vi "pop_integer_array.vi"(8 "error in (no error)":errorcluster, 11 "Lua in":refnum<class "Lua.lvclass">) -> (0 "error out":errorcluster, 2 "value":i64[](array[numeric]), 3 "Lua out":refnum<class "Lua.lvclass">)   [LabVIEW 2020, in "Lua for LabVIEW.lvlib" / "Lua.lvclass"]
doc: "Pop a numeric value from the stack."
uses:
  Lua.lvclass
  Lua.lvclass/Lua.ctl
  lib/lua.dll/lua.dll.lvlib
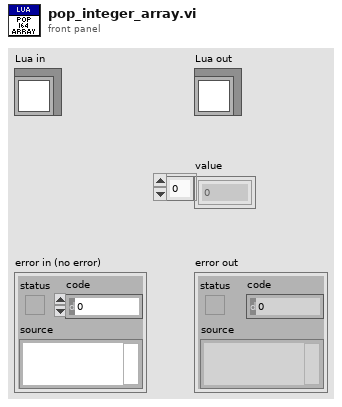
[diagram p1: front panel]
types:
  T1 = typedef "lua.dll.lvlib/lua_types.ctl" = i32
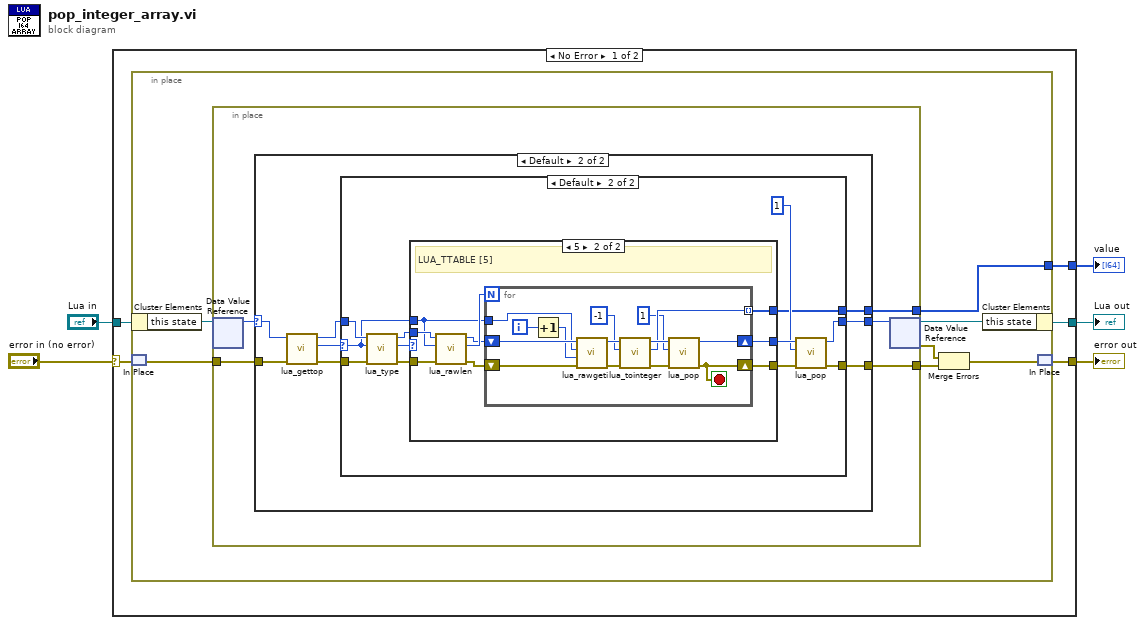
[diagram p0: block diagram]
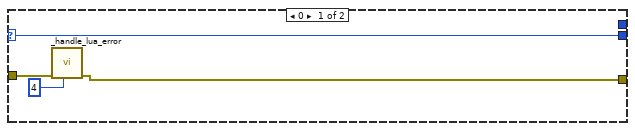
[diagram p2: hidden frame]
diagram:
  n1 = case shown="No Error" "error in (no error)" {
    selector: "error in (no error)" -> [w7 w75]
    tunnel: [w8 w75] -> w2
    tunnel: [w9 w74] -> w3
    tunnel: "Lua in" -> [w10 w74]
    tunnel: [w6 _] -> w1
    frame No Error {
      n2 = in-place {
        in-place-border: [w16] -> w6
        n3 = in-place-cluster #1(w10) -> ("this state"=w12:refnum<data-value>)
        n4 = in-place-match #2(w7) -> (w17:errorcluster)
        n5 = in-place {
          in-place-border: w17 -> [w22]
          in-place-border: [w21] -> w16
          in-place-border: [w20] -> w13
          n6 = in-place-dvr #3(w12) -> (w18:u64)  [unwired: 1 out]
          n7 = case shown="Default" w18 {
            selector: w18 -> [w26 w30]
            tunnel: [w26 w34] -> w19
            tunnel: w22 -> [w23 w31]
            tunnel: [w24 w33] -> w20
            tunnel: [_ w32] -> w21
            frame 0 {
              n8 = call "_handle_lua_error.vi"("lua status"=4 ("lua_load errcode"), "error in (no error)"=w23) -> ("error out"=w24:errorcluster)  [unwired: 9 in]
            }
            frame Default {
              n9 = call "lua_gettop.vi"("error in (no error)"=w31, "lua_state_p"=w30) -> ("error out"=w28:errorcluster, "index"=w27:i32, "lua_state_p out"=w29:u64)  [unwired: 7 in]
              n10 = case shown="Default" w27 {
                selector: w27 -> [_ w37]
                tunnel: [w36 w45] -> w34
                tunnel: [w35 w44] -> w33
                tunnel: [_ w40] -> w32
                tunnel: w29 -> [w36 w39]
                tunnel: w28 -> [w35 w38]
                frame 0 {
                }
                frame Default {
                  n11 = call "lua_type.vi"("error in (no error)"=w38, "index"=w37, "lua_state_p"=w39) -> ("error out"=w41:errorcluster, "lua type"=w48:T1, "lua_state_p out"=w47:u64)  [unwired: 6 in]
                  n12 = case shown="5" w48 {
                    tunnel: [w49 w52] -> w46
                    tunnel: w47 -> [w49 w59]
                    tunnel: [w50 w53] -> w42
                    tunnel: w41 -> [w50 w58]
                    tunnel: [_ w54] -> w40
                    tunnel: w37 -> [_ w51]
                    frame Default {
                    }
                    frame 5 {
                      # "LUA_TTABLE [5]"
                      n13 = call "lua_rawlen.vi"("error in (no error)"=w58, "index"=w51, "lua_state_p"=w59) -> ("error out"=w55:errorcluster, "length"=w57:u64, "lua_state_p out"=w56:u64)  [unwired: 6 in]
                      n14 = for {
                        N: w57 -> [_]
                        shift-right: [w64] -> w52
                        shift-left: w56 -> [w73]
                        shift-right: [w61] -> w53
                        shift-left: w55 -> [w68]
                        tunnel: [w65] -> w54 mode=indexing
                        tunnel: w51 -> [w60]
                        i -> [w72]
                        stop <- w61 stop-if-true
                        n15 = Increment(x=w72) -> (x+1=w71:i32)
                        n16 = call "lua_rawgeti.vi"("error in (no error)"=w68, "n"=w71, "index"=w60, "lua_state_p"=w73) -> ("error out"=w69:errorcluster, "lua_state_p out"=w70:u64)  [unwired: 5 in, 1 out]
                        n17 = call "lua_tointeger.vi"("error in (no error)"=w69, "index"=-1, "lua_state_p"=w70) -> ("error out"=w62:errorcluster, "integer"=w65:i64, "lua_state_p out"=w66:u64)  [unwired: 5 in, 1 out]
                        n18 = call "lua_pop.vi"("error in (no error)"=w62, "n"=1, "lua_state_p"=w66) -> ("error out"=w61:errorcluster, "lua_state_p out"=w64:u64)  [unwired: 7 in]
                      }
                    }
                  }
                  n19 = call "lua_pop.vi"("error in (no error)"=w42, "n"=1, "lua_state_p"=w46) -> ("error out"=w44:errorcluster, "lua_state_p out"=w45:u64)  [unwired: 7 in]
                }
              }
            }
          }
          n20 = in-place-dvr #3(w19) -> (w11:refnum<data-value>, w15:errorcluster)
        }
        n21 = Merge Errors(w15, w13) -> (w14:errorcluster)
        n22 = in-place-cluster #1("this state"=w11) -> (w9:refnum<class "Lua.lvclass">)
        n23 = in-place-match #2(w14) -> (w8:errorcluster)
      }
    }
    frame Error {
    }
  }
  "error out" <- w2
  "Lua out" <- w3
  "value" <- w1
